vi "ServerStop.vi"(8 "error in (no error)":errorcluster, 11 "TcpServer in":refnum<class "TcpServer.lvclass">) -> (0 "error out":errorcluster, 3 "TcpServer out":refnum<class "TcpServer.lvclass">)   [LabVIEW 2022 SP3, in "TcpServer.lvlib" / "TcpServer.lvclass"]
uses:
  TcpServer.lvclass
  C:/Users/jakub/repos/gh/sw4sys/lv-tcp-server-sample/LoggingActor/Source/LoggingActor/LoggingActor/LoggingActor.lvclass
  LoggingActor/Source/LoggingActor/LoggingActor/LoggingActor.lvclass/LoggingActor.ctl
  TcpServer.lvclass/TcpServer.ctl
  _ServerState.ctl
  <vilib>/ActorFramework/Time-Delayed Send Message/Time-Delay Override Options.ctl
  TcpSocket/Source/TcpSocket/TcpSocket/TcpSocket.lvclass/TcpSocket.ctl
  TcpSocket/Source/TcpSocket/TcpServer/TcpServer.lvclass/TcpServer.ctl
  TcpSocket/Source/TcpSocket/TcpSocket/Read Address.vi
  TcpSocket/Source/TcpSocket/TcpSocket/Read Port.vi
  TcpSocket/Source/TcpSocket/TcpSocket/Read Connection.vi
  TcpSocket/Source/TcpSocket/TcpSocket/Read ReadMode.vi
  TcpSocket/Source/TcpSocket/TcpSocket/Read OpenTimeout.vi
  TcpSocket/Source/TcpSocket/TcpSocket/Read ReadTimeout.vi
  TcpSocket/Source/TcpSocket/TcpSocket/Read WriteTimeout.vi
  TcpSocket/Source/TcpSocket/TcpServer/Read ConnectionTimeout.vi
  LoggingActor/Source/LoggingActor/LoggingActor/Read Logger.vi
  TcpSocket/Source/TcpSocket/TcpServer/TcpServer.lvclass
  C:/Users/jakub/repos/gh/sw4sys/lv-tcp-server-sample/TcpSocket/Source/TcpSocket/TcpSocket/TcpSocket.lvclass
  Logger/Source/Logger/Logger.lvclass
  <vilib>/ActorFramework/Actor/Actor.lvclass
  TcpServer Messages/KillAllConnections Msg/KillAllConnections Msg.lvclass
  C:/Program Files (x86)/National Instruments/LabVIEW 2022/vi.lib/ActorFramework/Actor/Actor.lvclass
  C:/Users/jakub/repos/gh/sw4sys/lv-tcp-server-sample/TcpServerSample/Source/TcpServer/TcpServer/TcpServer.lvclass
  C:/Users/jakub/repos/gh/sw4sys/lv-tcp-server-sample/TcpServerSample/Source/Connection/CallerMessage/CallerMessage.lvclass
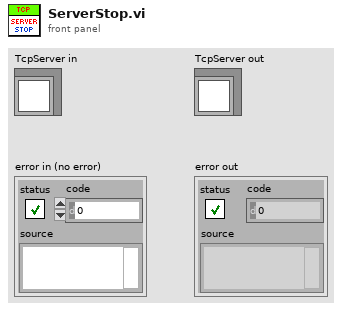
[diagram p1: front panel]
types:
  T1 = typedef "Time-Delay Override Options.ctl" = enum16{"Send next copy now", "Skip next scheduled copy", "Send next copy now and stop all further copies", "Stop all further copies"}
  T2 = typedef "TcpServer.lvlib/TcpServer.lvclass/_ServerState.ctl" = enum16{"Idle", "Running"}
  T3 = enum16{"Standard", "Buffered", "CRLF", "Immediate"}
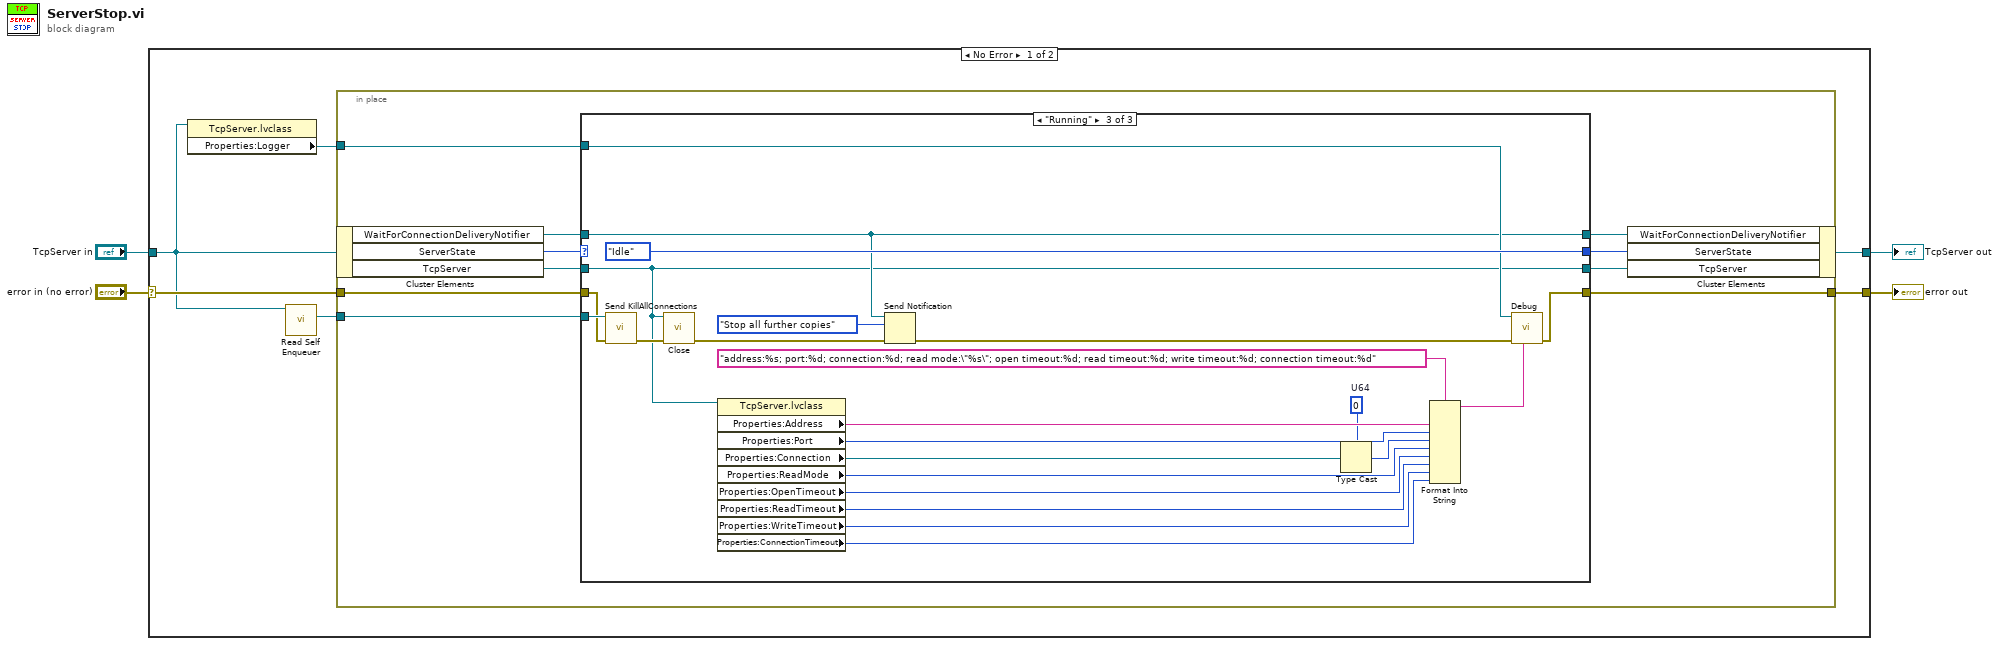
[diagram p0: block diagram]
diagram:
  n1 = case shown="No Error" "error in (no error)" {
    selector: "error in (no error)" -> [w10 w53]
    tunnel: [w7 w53] -> w2
    tunnel: [w8 w52] -> w1
    tunnel: "TcpServer in" -> [w6 w52]
    frame No Error {
      n2 = property class="TcpServer.lvclass"(reference=w6) -> ("Properties:Logger"=w9:refnum<class "Logger.lvclass">)  [unwired: 1 in, 2 out]
      n3 = call <vilib>:"Read Self Enqueuer.vi"("Actor"=w6) -> ("Self Enqueuer"=w5:refnum<class "Message Enqueuer.lvclass">)  [unwired: 10 in]
      n4 = in-place {
        in-place-border: [w20] -> w7
        in-place-border: w10 -> [w19]
        in-place-border: w9 -> [w14]
        in-place-border: w5 -> [w11]
        n5 = in-place-cluster #1(w6) -> ("WaitForConnectionDeliveryNotifier"=w13:refnum<notifier>, "ServerState"=w16:T2, "TcpServer"=w18:refnum<class "TcpServer.lvclass">)
        n6 = case shown="\"Running\"" w16 {
          selector: w16 -> [w22 w26 _]
          tunnel: [w23 w27 w38] -> w20
          tunnel: w19 -> [w23 w27 w32]
          tunnel: w18 -> [w24 w28 w31]
          tunnel: [w24 w28 w31] -> w17
          tunnel: [w22 w26 _ServerState."Idle" ("ServerState")] -> w15
          tunnel: w14 -> [_ _ w37]
          tunnel: w13 -> [w21 w25 w35]
          tunnel: [w21 w25 w35] -> w12
          tunnel: w11 -> [_ _ w34]
          frame Default {
          }
          frame "Idle" {
          }
          frame "Running" {
            w46 = u64 0  # U64
            n7 = call "Send KillAllConnections.vi"("error in (no error)"=w32, "Message Enqueuer"=w34) -> ("error out"=w33:errorcluster)  [unwired: 8 in, 1 out]
            n8 = call-dynamic "Close.vi"("error in (no error)"=w33, "TcpSocket in"=w31) -> ("error out"=w30:errorcluster)  [unwired: 9 in]
            n9 = property class="TcpServer.lvclass"(reference=w31) -> ("Properties:Address"=w50:string, "Properties:Port"=w49:u16, "Properties:Connection"=w48:refnum<k5>, "Properties:ReadMode"=w45:T3, "Properties:OpenTimeout"=w44:i32, "Properties:ReadTimeout"=w43:i32, "Properties:WriteTimeout"=w42:i32, "Properties:ConnectionTimeout"=w41:i32)  [unwired: 1 in, 2 out]
            n10 = Send Notification(notification=Time-Delay_Override_Options."Stop all further copies", notifier=w35, error in (no error)=w30) -> (error out=w29:errorcluster)  [unwired: 1 out]
            n11 = Type Cast(type=w46, x=w48) -> (*(type *) &x=w47:u64)
            n12 = Format Into String(format string="address:%s; port:%d; connection:%d; read mode:\"%s\"; open timeout:%d; read timeout:%d; write timeout:%d; connection timeout:%d", w50, w49, w47, w45, w44, w43, w42, w41) -> (resulting string=w39:string)  [unwired: 2 in, 1 out]
            n13 = call-dynamic "Debug.vi"("Message"=w39, "error in (no error)"=w29, "Logger in"=w37) -> ("error out"=w38:errorcluster)  [unwired: 5 in, 1 out]
          }
        }
        n14 = in-place-cluster #1("WaitForConnectionDeliveryNotifier"=w12, "ServerState"=w15, "TcpServer"=w17) -> (w8:refnum<class "TcpServer.lvclass">)
      }
    }
    frame Error {
    }
  }
  "error out" <- w2
  "TcpServer out" <- w1
